vi "OCR SubVI.vi"(8 "error in (no error)":errorcluster, 10 "ROI Array Within Image":T1[](array[typedef]) {"Contours"."Type" items=["No Selection", "Point", "Line", "Rectangle", "Oval", "Polygon", "Freehand Region", "Annulus", "Unused2", "Unused3", "Broken Line", "Freehand Line", "Rotated Rectangle"]}, 11 "Refnum in":T2) -> (0 "error out":errorcluster, 2 "Read String":string[](array[string]), 3 "Image Out Ref":T2)   [LabVIEW 2014]
doc: "This subVI takes in an array of ROI descriptions, and performs OCR (Optical Character Recognition). It outputs the string of characters found within the ROIs."
uses:
  <vilib>/vision/Image Controls.llb/IMAQ Image.ctl
  <vilib>/vision/NI_Vision_Development_Module.lvlib
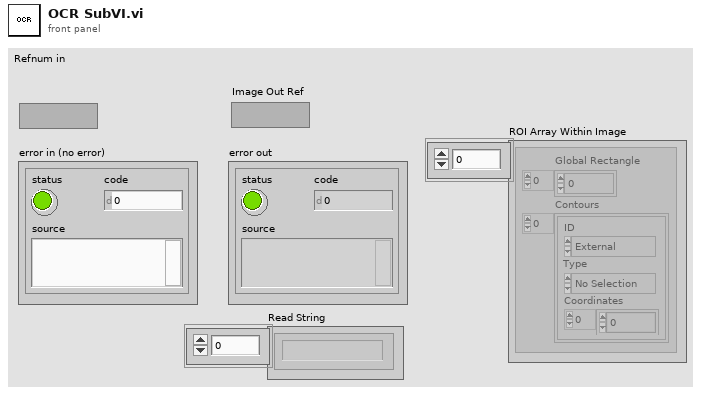
[diagram p1: front panel]
types:
  T1 = typedef "ROI Descriptor" = cluster{"Global Rectangle":i32[], "Contours":cluster{"ID":enum32{"External", "Internal"}, "Type":u32, "Coordinates":i32[]}[]}
  T2 = typedef "IMAQ Image.ctl" = refnum<image>
  T3 = cluster{"Threshold Data":cluster{"Method":enum16{"Fixed Range", "Uniform", "Linear", "Non Linear", "Local", "Color"}, "Looking for":u32, "Color Mode":u32, "Kernel Size":cluster{"Width":i32, "Height":i32}, "Ranges":cluster{"Min":i32, "Max":i32}[]}, "Reject Border":bool, "Number Of Erosions":i32, "Size & Spacing":cluster{"Segment Algorithm":u16, "Min Bounding Rect Width":i32, "Max Bounding Rect Width":i32, "Min Bounding Rect Height":i32, "Max Bounding Rect Height":i32, "Min Character Size":i32, "Max Character Size":i32, "Min Char Spacing":i32, "Max Horiz Element Spacing":i32, "Max Vert Element Spacing":i32, "Max Space Distance":i32}, "Read Options":cluster{"Read Strategy":i32, "Read Resolution":i32, "Scale Dependant":bool, "Aspect Ratio":i32, "Acceptance Level":i32, "Substitution Character":string, "MultiLine":bool}, "Valid Characters":cluster{"Pre-defined characters":i32, "User-defined characters":string}[], "Use Text Pattern":bool, "Orientation":u32, "# Lines Expected":u32, "Number of Blocks":i32}
  T4 = typedef "IMAQ OCR Session.ctl" = refnum<k1>
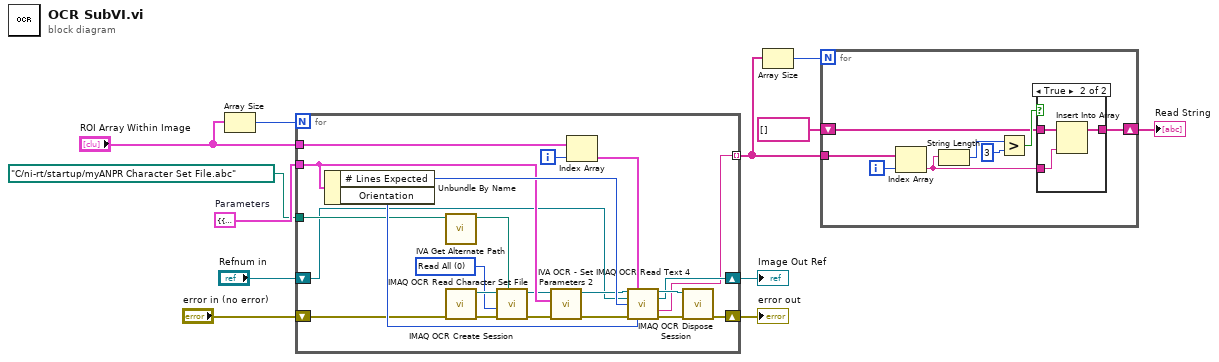
[diagram p0: block diagram]
diagram:
  w12 = T3 {"Threshold Data"={"Method"=enum."Fixed Range", "Looking for"=0, "Color Mode"=0, "Kernel Size"={"Width"=32, "Height"=32}, "Ranges"=[{"Min"=1, "Max"=255}]}, "Reject Border"=TRUE, "Number Of Erosions"=0, "Size & Spacing"={"Segment Algorithm"=0, "Min Bounding Rect Width"=1, "Max Bounding Rect Width"=800, "Min Bounding Rect Height"=10, "Max Bounding Rect Height"=800, "Min Character Size"=20, "Max Character Size"=65536, "Min Char Spacing"=1, "Max Horiz Element Spacing"=1, "Max Vert Element Spacing"=0, "Max Space Distance"=65536}, "Read Options"={"Read Strategy"=0, "Read Resolution"=2, "Scale Dependant"=FALSE, "Aspect Ratio"=400, "Acceptance Level"=700, "Substitution Character"="?", "MultiLine"=TRUE}, "Valid Characters"=[], "Use Text Pattern"=FALSE, "Orientation"=0, "# Lines Expected"=0, "Number of Blocks"=4}  # Parameters
  n1 = Array Size(array="ROI Array Within Image") -> (size(s)=w6:i32)
  n2 = for {
    N: w6 -> [_]
    tunnel: w12 -> [w30]
    tunnel: path "C:/ni-rt/startup/myANPR Character Set File.abc" ("File Path") -> [w28]
    shift-right: [w25] -> w9
    shift-left: "error in (no error)" -> [w29]
    shift-right: [w23] -> w7
    shift-left: "Refnum in" -> [w24]
    tunnel: "ROI Array Within Image" -> [w22]
    tunnel: [w19] -> w2 mode=indexing
    i -> [w21]
    w16 = 0 items=["Read All", "Read Character Set Only", "Read Properties Only"] ("Read Options")
    n3 = Unbundle By Name(w30) -> ("# Lines Expected"=w34:u32, "Orientation"=w33:u32)
    n4 = call <vilib>:"IVA Get Alternate Path.vi"("Path In"=w28) -> ("Path Out"=w14:path)  [unwired: 10 out]
    n5 = call "IMAQ OCR Create Session"("error in (no error)"=w29) -> ("error out"=w17:errorcluster, "IMAQ OCR Session"=w18:T4)  [unwired: 9 out]
    n6 = call "IMAQ OCR Read Character Set File"("File Path"=w14, "error in (no error)"=w17, "Read Options"=w16, "IMAQ OCR Session"=w18) -> ("error out"=w15:errorcluster, "IMAQ OCR Session (dup)"=w13:T4)  [unwired: 1 in, 5 out]
    n7 = call <vilib>:"IVA OCR - Set Parameters 2.vi"("error in (no error)"=w15, "Parameters"=w30, "IMAQ OCR Session"=w13) -> ("error out"=w31:errorcluster, "IMAQ OCR Session Out"=w32:T4)  [unwired: 7 in]
    n8 = Index Array(array=w22, index=w21) -> (element=w20:T1)
    n9 = call "IMAQ OCR Read Text 4"("IMAQ OCR Session"=w32, "ROI Descriptor"=w20, "Image"=w24, "Number of Lines Requested"=w34, "error in (no error)"=w31, "Orientation"=w33) -> ("IMAQ OCR Session (dup)"=w26:T4, "Image (dup)"=w23:T2, "Read String"=w19:string, "error out"=w27:errorcluster)  [unwired: 6 out]
    n10 = call "IMAQ OCR Dispose Session"("error in (no error)"=w27, "IMAQ OCR Session"=w26) -> ("error out"=w25:errorcluster)  [unwired: 9 in]
  }
  "error out" <- w9
  "Image Out Ref" <- w7
  n11 = Array Size(array=w2) -> (size(s)=w3:i32)
  n12 = for {
    N: w3 -> [_]
    tunnel: w2 -> [w42]
    shift-right: [w35] -> w1
    shift-left: string[] [] -> [w37]
    i -> [w41]
    n13 = Index Array(array=w42, index=w41) -> (element=w36:string)
    n14 = String Length(string=w36) -> (length=w40:i32)
    n15 = Greater?(x=w40, y=3) -> (0:w38:bool)
    n16 = case shown="True" w38 {
      tunnel: w37 -> [_ w45]
      tunnel: w36 -> [_ w44]
      tunnel: [_ w43] -> w35
      frame False {
      }
      frame True {
        n17 = Insert Into Array(array=w45, new element=w44) -> (w43:string[])  [unwired: 1 in]
      }
    }
  }
  "Read String" <- w1
